vi "Select Review Frame.vi"(8 "RevFrame":i32, 9 "PI pos (um) in":dbl[](array[numeric]), 10 "dts":u64[](array[numeric]), 11 "Time (s) in":dbl[](array[numeric])) -> (1 "Position (um)":dbl=49.99, 2 "dt (ms)":u32, 3 "Time (s) out":dbl)   [LabVIEW 2020]
uses:
  _Globals/Global Controls.vi
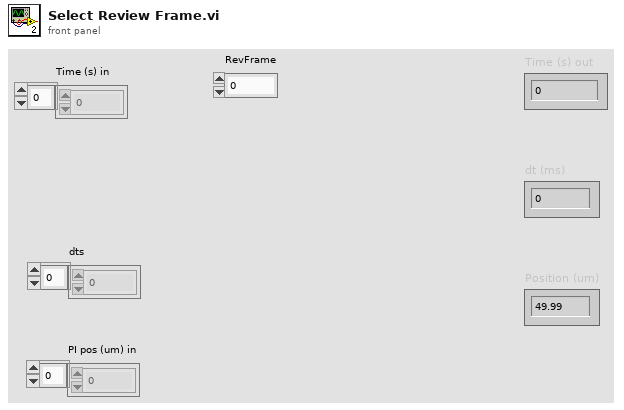
[diagram p1: front panel]
types:
  T1 = typedef "Review Ctrl Refs.ctl" = cluster{"RevFrame":refnum<vi>, "PIFOC Positions":refnum<vi>, "dts (ms)":refnum<vi>}
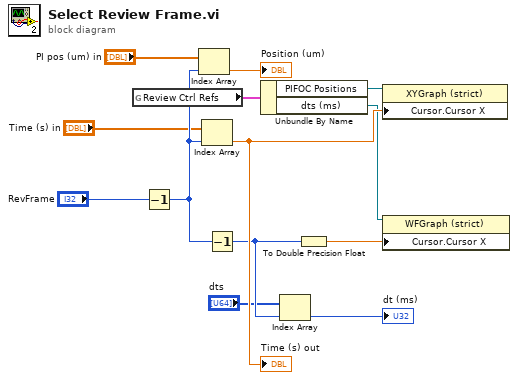
[diagram p0: block diagram]
diagram:
  n1 = global read "Global Controls.vi" "Review Ctrl Refs"() -> (w3:T1)
  n2 = Decrement(x="RevFrame") -> (x-1=w10:i32)
  n3 = Index Array(array="PI pos (um) in", index=w10) -> (element=→"Position (um)":dbl)
  n4 = Index Array(array="Time (s) in", index=w10) -> (element=w13:dbl)
  "Time (s) out" <- w13
  n5 = Decrement(x=w10) -> (x-1=w11:i32)
  n6 = Unbundle By Name(w3) -> ("PIFOC Positions"=w2:refnum<vi>, "dts (ms)"=w1:refnum<vi>)
  n7 = Index Array(array="dts", index=w11) -> (element=→"dt (ms)":u64)
  n8 = To Double Precision Float(number=w11) -> (double precision float=w8:dbl)
  n9 = property on="Property Node" class="XYGraph (strict)"(reference=w2, "Cursor.Cursor X"=w13) -> ()  [unwired: 1 in, 2 out]
  n10 = property on="Property Node" class="WFGraph (strict)"(reference=w1, "Cursor.Cursor X"=w8) -> ()  [unwired: 1 in, 2 out]
